vi "TrueFalseToBool.vi"(1 "String":string) -> (0 "Boolean":bool)   [LabVIEW 2017, in "GPString.lvlib"]
doc: "Converts the <B>String</B> input value to a True or False <B>Boolean</B>.\n\n\"TRUE\", \"YES\", \"T\", \"Y\", as well as any string representation of an integer number other than zero, yields a True <B>Boolean</B> output. Any other <B>String</B> yields a False <B>Boolean</B> output. The match is case-insensitive.\n\nThis VI is inlined.\n\nSteen Schmidt\nGPower\n24/1 2013"
uses:
  GPString.lvlib
panel:
  # "Copyright © 2013\nSteen Schmidt, GPower\nSee enclosed license file for terms and conditions"
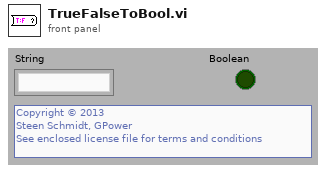
[diagram p1: front panel]
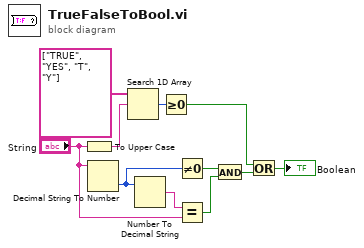
[diagram p0: block diagram]
diagram:
  n1 = To Upper Case(1:"String") -> (0:w11:string)
  n2 = Decimal String To Number(string="String") -> (number=w10:i32)  [unwired: 3 out]
  n3 = Search 1D Array(1D array=string[] ["TRUE", "YES", "T", "Y"], element=w11) -> (index of element=w8:i32)  [unwired: 1 out]
  n4 = Number To Decimal String(number=w10) -> (decimal integer string=w5:string)  [unwired: 1 out]
  n5 = Greater Or Equal To 0?(x=w8) -> (x >= 0?=w2:bool)
  n6 = Not Equal To 0?(x=w10) -> (x != 0?=w9:bool)
  n7 = Equal?(x=w5, y="String") -> (x = y?=w3:bool)
  n8 = And(x=w9, y=w3) -> (x .and. y?=w1:bool)
  n9 = Or(x=w2, y=w1) -> (x .or. y?=→"Boolean":bool)
